vi "Save Channel Info.vi"(6 "Sample rate":sgl format="%.2f", 8 "error in":errorcluster, 9 "time":dbl format="%.2f", 10 "channel info":T1(array[cluster]) {"sensor sensitivity (mV/EU)" format="%.2f"; "offset" format="%.2f"; "multiplier" format="%.2f"}, 11 "refnum in":refnum<file>) -> (0 "error out":errorcluster, 3 "refnum out":refnum<file>)   [LabVIEW 2017]
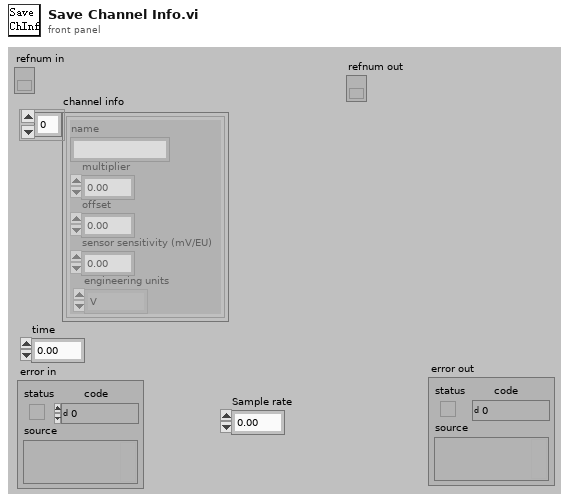
[diagram p1: front panel]
types:
  T1 = cluster{"name":string, "multiplier":sgl, "offset":sgl, "sensor sensitivity (mV/EU)":dbl, "engineering units":enum16{"custom...", "V", "Pa", "g", "m/s^2", "m/s", "m", "in/s^2", "in/s", "in"}}[]
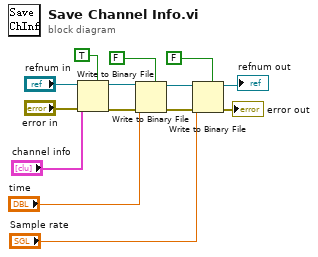
[diagram p0: block diagram]
diagram:
  n1 = Write to Binary File(file (use dialog)="refnum in", data="channel info", error in="error in", 5:TRUE ("header (F)")) -> (refnum out=w12:refnum<file>, error out=w13:errorcluster)  [unwired: 2 in, 1 out]
  n2 = Write to Binary File(file (use dialog)=w12, data="time", error in=w13, 5:FALSE ("prepend array or string size? (T)")) -> (refnum out=w11:refnum<file>, error out=w10:errorcluster)  [unwired: 2 in, 1 out]
  n3 = Write to Binary File(file (use dialog)=w11, data="Sample rate", error in=w10, 5:FALSE ("prepend array or string size? (T)")) -> (refnum out=→"refnum out":refnum<file>, error out=→"error out":errorcluster)  [unwired: 2 in, 1 out]
